vi "Timing Test using timed control loop with DAQ trig src.vi"() -> ()   [LabVIEW 2022 SP3]
uses:
  <vilib>/Utility/error.llb/DialogType.ctl
  <vilib>/Platform/TimedLoop/XDataNode/timing_clust.ctl
  <vilib>/Platform/TimedLoop/XDataNode/nitl_modes.ctl
  <vilib>/Platform/TimedLoop/XDataNode/wakeup.ctl
  <vilib>/Platform/TimedLoop/XDataNode/XDataNode.xnode
  <resource>/objmgr/daqmx.rc
  <vilib>/Platform/TimedLoop/XDataNode/XDNodeRunTimeDep.lvlib
panel:
  in  "stop":bool
  out "elapsed":dbl
  out "fs":dbl
  out "elapsed time":dbl
  in  "DAQmx Task Name":refnum<k21>="DopplerI"
  out "num iter 2":i32
  in  "Numeric":i32
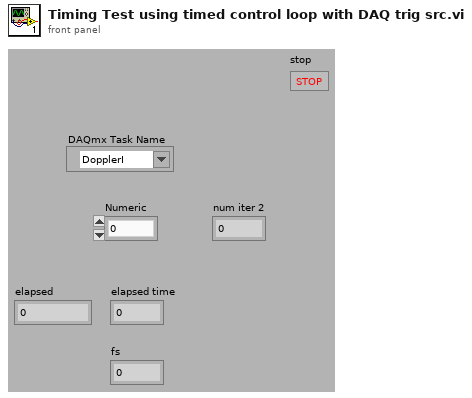
[diagram p1: front panel]
types:
  T1 = typedef "DialogType.ctl" = u16
  T2 = typedef "XDNodeRunTimeDep.lvlib/timing_clust.ctl" = cluster{"Expected End [f-1]":u64, "Actual End [f-1]":u64, "Finished Late? [f-1]":bool, "Expected End [i-1]":u64, "Actual End [i-1]":u64, "Finished Late? [i-1]":bool, "Expected Start [i]":u64, "Actual Start [i]":u64, "Expected Start [f]":u64, "Actual Start [f]":u64, "Source Name":string, "Structure Name":string, "Period":i64, "Deadline":i64, "Offset":i64, "Start":i64, "Priority":i32, "Timeout":i32, "Mode":T3, "Wakeup Reason":T4, "Error":errorcluster, "Source Type":string, "Secondary Source Type":string, "Global End Time":u64, "Global Start Time":u64, "Frame Duration":u64, "Iteration Duration":u64, "Assigned CPU":i32, "I/O Scan Engine Mode":u32}
  T3 = typedef "XDNodeRunTimeDep.lvlib/nitl_modes.ctl" = enum32{"No Change", "Process missed periods, maintain original phase", "Discard missed periods, maintain original phase", "Process missed periods, ignore original phase", "Discard missed periods, ignore original phase"}
  T4 = typedef "XDNodeRunTimeDep.lvlib/wakeup.ctl" = enum32{"Normal", "Aborted", "Asynchronous wakeup", "Timing source error", "Timed loop error", "Timeout"}
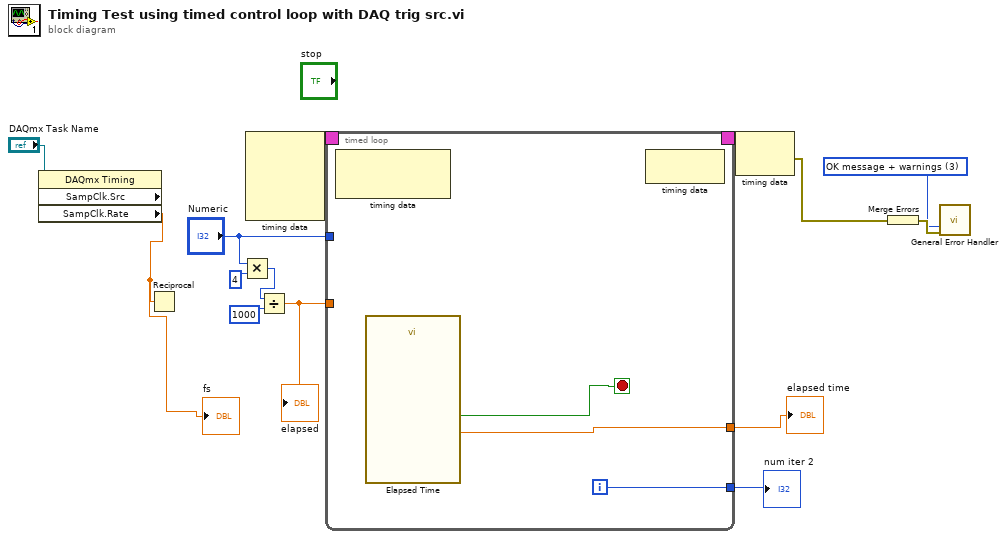
[diagram p0: block diagram]
diagram:
  w3 = T1 3 items=["no dialog", "OK message", "continue or stop message", "OK message + warnings", "continue/stop + warnings"] ("type of dialog (OK msg:1)")
  n1 = property class="DAQmx Timing" props=["SampClk.Src", "SampClk.Rate"](reference="DAQmx Task Name") -> ("SampClk.Rate"=w9:dbl)  [unwired: 1 in, 3 out]
  "fs" <- w9
  n2 = Reciprocal(x=w9) -> ()  [unwired: 1 out]
  n3 = Multiply(x="Numeric", y=4) -> (x*y=w6:i32)
  n4 = node-c288() -> (w13:T2)  [unwired: 4 out]
  n5 = Divide(x=w6, y=1000) -> (x/y=w8:dbl)
  "elapsed" <- w8
  n6 = timed-loop {
    tunnel: "Numeric" -> [_]
    tunnel: w8 -> [_]
    tunnel: [w15] -> w14
    timing: w13 -> [_]
    timing-out: [_] -> w12
    tunnel: [w16] -> w10
    i -> [w15]
    stop <- w17 stop-if-true
    n7 = node-c288() -> ()  [unwired: 3 out]
    n8 = call "Elapsed Time"() -> ("Elapsed Time (s)"=w16:dbl, "Time has Elapsed"=w17:bool)  [unwired: 5 in, 13 out]
    n9 = node-c288() -> ()  [unwired: 2 out]
  }
  "num iter 2" <- w14
  "elapsed time" <- w10
  n10 = node-c288(w12) -> (w2:errorcluster)
  n11 = Merge Errors(w2) -> (w4:errorcluster)
  n12 = call <vilib>:"General Error Handler.vi"("type of dialog (OK msg:1)"=w3, "error in (no error)"=w4) -> ()  [unwired: 1 in, 13 out]
